vi "random_fill.vi"(8 "error in (no error)":errorcluster, 9 "minimum value":dbl, 10 "maximum value":dbl=1.0, 11 "Image in":refnum<class "Image.lvclass">) -> (0 "error out":errorcluster, 3 "Image out":refnum<class "Image.lvclass">)   [LabVIEW 2010, in "Image.lvclass"]
uses:
  Image.lvclass
  storage_mode.ctl
  error_codes_ring.ctl
  ErrorController/ErrorController/class_data.vi
  ErrorController/ErrorController/ErrorController.lvclass
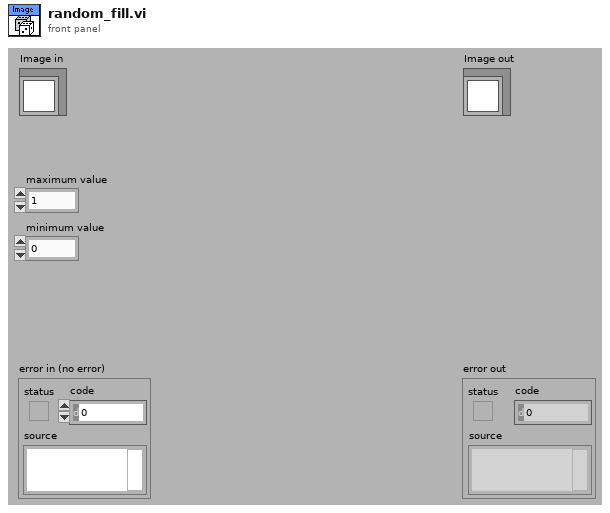
[diagram p1: front panel]
types:
  T1 = typedef "Image.lvclass/storage_mode.ctl" = enum16{"RAM", "disk"}
  T2 = typedef "Image Type" = u32
  T3 = typedef "IMAQ Image.ctl" = refnum<image>
  T4 = typedef "Image.lvclass/error_codes_ring.ctl" = u16
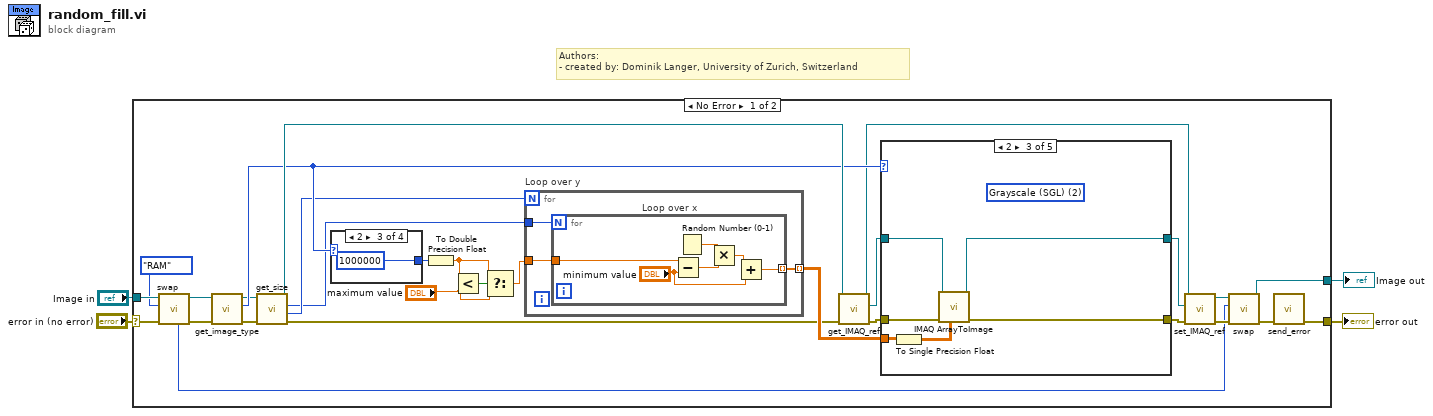
[diagram p0: block diagram]
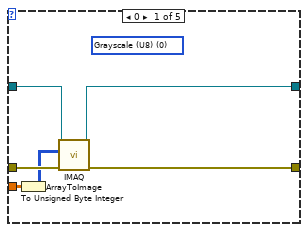
[diagram p2: hidden frame]
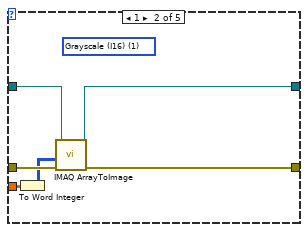
[diagram p3: hidden frame]
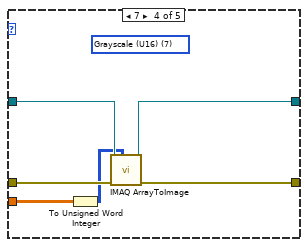
[diagram p4: hidden frame]
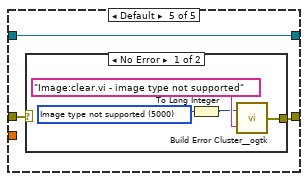
[diagram p5: hidden frame]
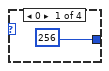
[diagram p7: hidden frame]
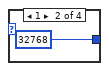
[diagram p8: hidden frame]
diagram:
  # "Authors: \n- created by: Dominik Langer, University of Zurich, Switzerland"
  n1 = case shown="No Error" "error in (no error)" {
    selector: "error in (no error)" -> [w22 w79]
    tunnel: [w5 w79] -> w3
    tunnel: [w15 w78] -> w1
    tunnel: "Image in" -> [w24 w78]
    frame No Error {
      n2 = call-dynamic "swap.vi"("error in (no error)"=w22, "storage type target"=storage_mode."RAM", "Image in"=w24) -> ("error out"=w21:errorcluster, "Image out"=w23:refnum<class "Image.lvclass">, "previous storage mode"=w13:T1)  [unwired: 6 out]
      n3 = call-dynamic "get_image_type.vi"("error in (no error)"=w21, "Image.lvclass in"=w23) -> ("error out"=w27:errorcluster, "Image Type"=w26:T2, "Image.lvclass out"=w25:refnum<class "Image.lvclass">)  [unwired: 7 out]
      n4 = call-dynamic "get_size.vi"("error in (no error)"=w27, "Image in"=w25) -> ("error out"=w32:errorcluster, "y resolution"=w12:i32, "x resolution"=w11:i32, "Image out"=w30:refnum<class "Image.lvclass">)  [unwired: 6 out]
      n5 = case shown="2" w26 {
        tunnel: [256 32768 1000000 _] -> w28
        frame 0 {
        }
        frame 1 {
        }
        frame 2 {
        }
        frame Default {
        }
      }
      n6 = To Double Precision Float(number=w28) -> (double precision float=w8:dbl)
      n7 = Less?(x=w8, y="maximum value") -> (x < y?=w10:bool)
      n8 = Select(t=w8, s=w10, f="maximum value") -> (s? t:f=w9:dbl)
      n9 = for "Loop over y" {
        N: w12 -> [_]
        tunnel: w11 -> [w71]
        tunnel: [w70] -> w33 mode=indexing
        tunnel: w9 -> [w69]
        n10 = for "Loop over x" {
          N: w71 -> [_]
          tunnel: [w72] -> w70 mode=indexing
          tunnel: w69 -> [w75]
          n11 = Subtract(x=w75, y="minimum value") -> (x-y=w76:dbl)
          n12 = Random Number (0-1)() -> (number: 0 to 1=w77:dbl)
          n13 = Multiply(x=w77, y=w76) -> (x*y=w74:dbl)
          n14 = Add(x=w74, y="minimum value") -> (x+y=w72:dbl)
        }
      }
      n15 = call-dynamic "get_IMAQ_ref.vi"("error in (no error)"=w32, "Image.lvclass in"=w30) -> ("error out"=w31:errorcluster, "Image"=w29:T3, "Image.lvclass out"=w16:refnum<class "Image.lvclass">)  [unwired: 7 out]
      n16 = case shown="2" w26 {
        tunnel: w33 -> [w36 w42 w51 w52 _]
        tunnel: [w37 w45 w50 w56 w59] -> w20
        tunnel: w31 -> [w39 w44 w49 w57 w60]
        tunnel: w29 -> [w38 w43 w48 w55 w58]
        tunnel: [w34 w40 w46 w54 w58] -> w19
        frame 0 {
          (unwired) T2 0 items=["Grayscale (U8)", "Grayscale (I16)", "Grayscale (SGL)", "Complex (CSG)", "RGB (U32)", "HSL (U32)", "RGB (U64)", "Grayscale (U16)"] ("Image Type")
          n17 = To Unsigned Byte Integer(number=w36) -> (unsigned 8bit integer=w35:u8[][])
          n18 = call "IMAQ ArrayToImage"("error in (no error)"=w39, "Image Pixels (U8)"=w35, "Image"=w38) -> ("error out"=w37:errorcluster, "Image Out"=w34:T3)  [unwired: 3 in, 4 out]
        }
        frame 1 {
          (unwired) T2 1 items=["Grayscale (U8)", "Grayscale (I16)", "Grayscale (SGL)", "Complex (CSG)", "RGB (U32)", "HSL (U32)", "RGB (U64)", "Grayscale (U16)"] ("Image Type")
          n19 = To Word Integer(number=w42) -> (16bit integer=w41:i16[][])
          n20 = call "IMAQ ArrayToImage"("error in (no error)"=w44, "Image Pixels (I16)"=w41, "Image"=w43) -> ("error out"=w45:errorcluster, "Image Out"=w40:T3)  [unwired: 3 in, 4 out]
        }
        frame 2 {
          (unwired) T2 2 items=["Grayscale (U8)", "Grayscale (I16)", "Grayscale (SGL)", "Complex (CSG)", "RGB (U32)", "HSL (U32)", "RGB (U64)", "Grayscale (U16)"] ("Image Type")
          n21 = To Single Precision Float(number=w51) -> (single precision float=w47:sgl[][])
          n22 = call "IMAQ ArrayToImage"("Image Pixels (Float)"=w47, "error in (no error)"=w49, "Image"=w48) -> ("error out"=w50:errorcluster, "Image Out"=w46:T3)  [unwired: 3 in, 4 out]
        }
        frame 7 {
          (unwired) T2 7 items=["Grayscale (U8)", "Grayscale (I16)", "Grayscale (SGL)", "Complex (CSG)", "RGB (U32)", "HSL (U32)", "RGB (U64)", "Grayscale (U16)"] ("Image Type")
          n23 = To Unsigned Word Integer(number=w52) -> (unsigned 16bit integer=w53:u16[][])
          n24 = call "IMAQ ArrayToImage"("Image Pixels (U16)"=w53, "error in (no error)"=w57, "Image"=w55) -> ("error out"=w56:errorcluster, "Image Out"=w54:T3)  [unwired: 3 in, 4 out]
        }
        frame Default {
          n25 = case shown="No Error" w60 {
            selector: w60 -> [_ w65]
            tunnel: [w64 w65] -> w59
            frame No Error {
              w62 = T4 5000 items=["Image type not supported"=5000] ("Ring")
              n26 = To Long Integer(number=w62) -> (32bit integer=w61:i32)
              n27 = call <userlib>:"Build Error Cluster__ogtk.vi"("String to Prepend to source (\"\")"="Image:clear.vi - image type not supported" ("String to Prepend to source (\"\")"), "code"=w61) -> ("error out"=w64:errorcluster)
            }
            frame Error {
            }
          }
        }
      }
      n28 = call-dynamic "set_IMAQ_ref.vi"("error in (no error)"=w20, "Image"=w19, "Image.lvclass in"=w16) -> ("error out"=w18:errorcluster, "Image.lvclass out"=w17:refnum<class "Image.lvclass">)  [unwired: 7 out]
      n29 = call-dynamic "swap.vi"("error in (no error)"=w18, "storage type target"=w13, "Image in"=w17) -> ("error out"=w6:errorcluster, "Image out"=w15:refnum<class "Image.lvclass">)  [unwired: 7 out]
      n30 = call "send_error.vi"("error in (no error)"=w6) -> ("error out"=w5:errorcluster)  [unwired: 10 in]
    }
    frame Error {
    }
  }
  "error out" <- w3
  "Image out" <- w1
